vi "Elevator_Execute.vi"() -> ()   [LabVIEW 2019]
uses:
  Globals/Climb_Globals.vi
  <vilib>/Rock Robotics/WPI/ThirdParty/Phoenix-LabVIEW/Motor Controller/Controls/CTRE_Phoenix_MotorControl_ControlMode.ctl
  Globals/Sensor_Values.vi
  Globals/Solenoid Globals.vi
  <vilib>/Rock Robotics/WPI/Solenoid/WPI_SolenoidValue.ctl
  <vilib>/Rock Robotics/WPI/Solenoid/WPI_SolenoidSetEnum.vi
panel:
  in  "BrakeDelay(ms)":u32
  in  "acceptable_error":dbl
  out "Waveform Chart":dbl(graph)
  out "Left_Value_Added":dbl
  out "Right_Value_Added":dbl
  out "difference(left-right)":dbl
  out "Left_Side_Input":dbl
  out "Right_Side_Input":dbl
  in  "Left Down %V P-Gain":dbl=0.0003
  in  "Right Down %V P-Gain":dbl=0.0003
  in  "Left SpeedControl P-Gain":dbl
  in  "Right SpeedControl P-Gain":dbl
  in  "Max_Elevator_Speed":dbl
  in  "Left Up %V P-Gain":dbl=0.0003
  in  "Right Up %V P-Gain":dbl=0.0003
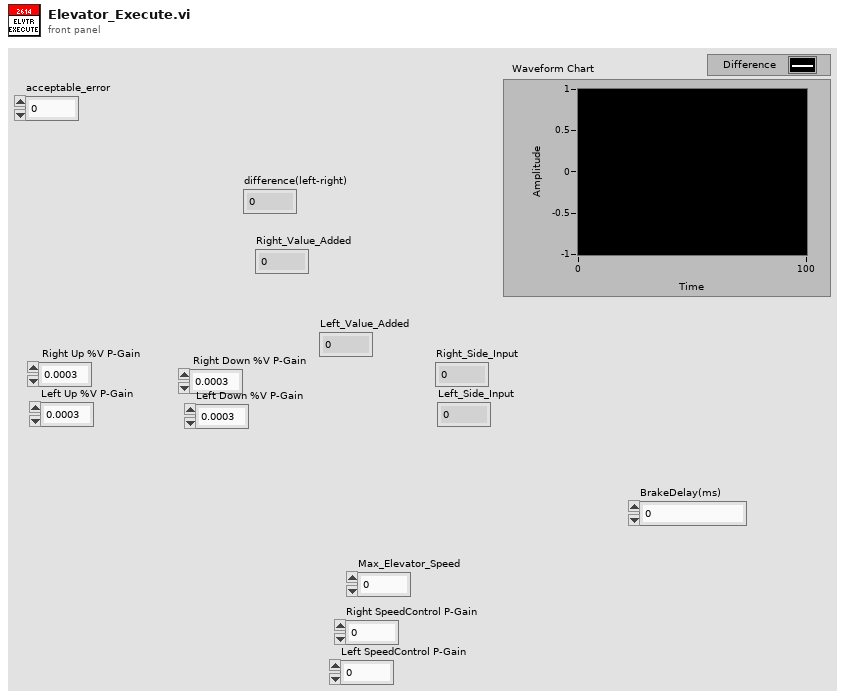
[diagram p1: front panel]
types:
  T1 = typedef "WPI_MotorControlDeviceRef.ctl" = cluster{"DeviceStatus":errorcluster, "Type":T2, "PWM":cluster{"PWM Channel":T3, "DeadBand":T4}, "CAN":cluster{"Device Number":u8, "SetOutput VI Ref":variant, "GetOutput VI Ref":variant, "Enable VI Ref":variant, "Disable VI Ref":variant, "Data":variant}, "Invert":bool, "DIO PWM":cluster{"PWM \"Enable\" Channel":T3, "DIOChannel":T5, "PWM Rate":dbl}}
  T2 = typedef "WPI_MotorControlType.ctl" = enum16{"PWM", "CAN", "DIO PWM"}
  T3 = typedef "FPGA_DIOPWMChannel.ctl" = enum8{"PWM 0", "PWM 1", "PWM 2", "PWM 3", "PWM 4", "PWM 5", "PWM 6", "PWM 7", "PWM 8", "PWM 9", "PWM MXP 0", "PWM MXP 1", "PWM MXP 2", "PWM MXP 3", "PWM MXP 4", "PWM MXP 5", "PWM MXP 6", "PWM MXP 7", "PWM MXP 8", "PWM MXP 9", "Invalid"}
  T4 = typedef "WPI_PWMDeadband.ctl" = cluster{"Name":string, "maxPositivePwm":i32, "minPositivePwm":i32, "centerPwm":i32, "maxNegativePwm":i32, "minNegativePwm":i32, "angularRange":u16}
  T5 = typedef "FPGA_DIOChannel.ctl" = enum8{"DIO 0", "DIO 1", "DIO 2", "DIO 3", "DIO 4", "DIO 5", "DIO 6", "DIO 7", "DIO 8", "DIO 9", "DIO MXP 0", "DIO MXP 1", "DIO MXP 2", "DIO MXP 3", "DIO MXP 4", "DIO MXP 5", "DIO MXP 6", "DIO MXP 7", "DIO MXP 8", "DIO MXP 9", "DIO MXP 10", "DIO MXP 11", "DIO MXP 12", "DIO MXP 13", "DIO MXP 14", "DIO MXP 15", "SPI Port CS1", "SPI Port CS2", "SPI Port CS3", "SPI Port MISO", "SPI Port MOSI", "Invalid"}
  T6 = typedef "WPI_SolenoidDevRef.ctl" = cluster{"DevStatus":errorcluster, "Pneumatics Control Module":u8, "Forward Solenoid Channel":T7, "Reverse Solenoid Channel":T7}
  T7 = typedef "WPI_SolenoidChannel.ctl" = enum8{"Solenoid 0", "Solenoid 1", "Solenoid 2", "Solenoid 3", "Solenoid 4", "Solenoid 5", "Solenoid 6", "Solenoid 7", "Invalid"}
  T8 = typedef "WPI_SolenoidValue.ctl" = enum16{"Off", "On", "Forward", "Reverse"}
  T9 = typedef "Climb_Elevator_Cluster.ctl" = cluster{"Extend?":bool, "Elevator_Throttle":dbl, "Control_States":T10}
  T10 = typedef "Climb_Elevator_Control_States.ctl" = enum16{"No-Op", "Brake", "Going_Up", "Going_Down", "Manual_PercentVoltage", "Manual_SpeedControl"}
  T11 = typedef "CTRE_Phoenix_MotorControl_ControlMode.ctl" = u16
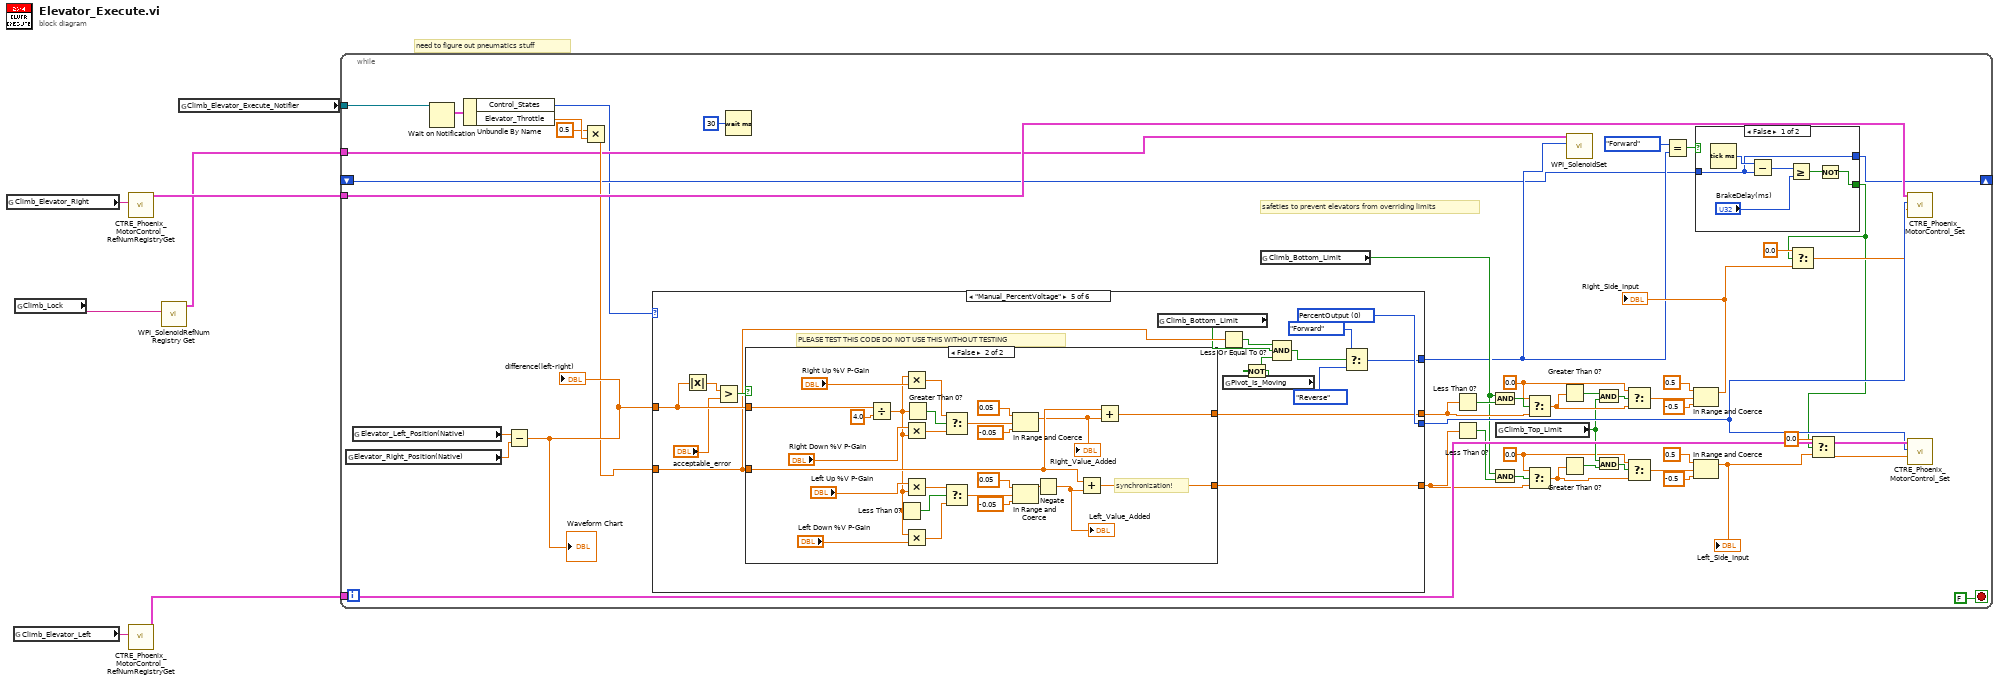
[diagram p0: block diagram]
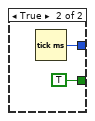
[diagram p2: hidden frame]
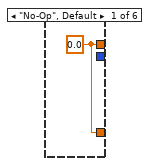
[diagram p3: hidden frame]
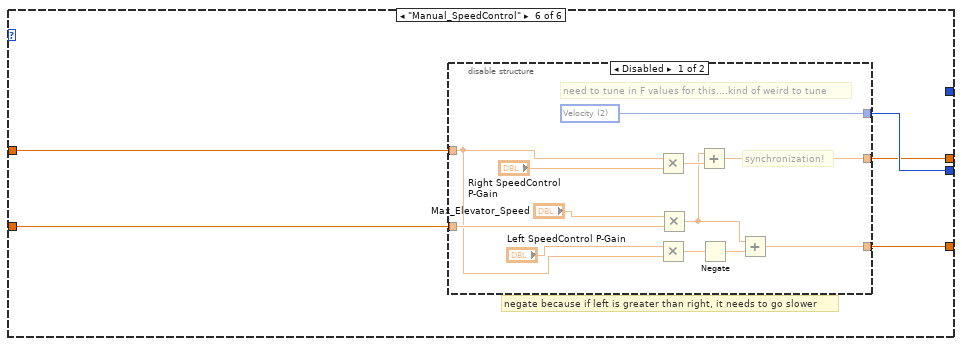
[diagram p8: hidden frame]
diagram:
  # "need to figure out pneumatics stuff"
  n1 = global read "Climb_Globals.vi" "Climb_Elevator_Right"() -> (w4:string)
  n2 = global read "Climb_Globals.vi" "Climb_Elevator_Left"() -> (w3:string)
  n3 = global read "Solenoid Globals.vi" "Climb_Lock"() -> (w2:string)
  n4 = call <vilib>:"CTRE_Phoenix_MotorControl_RefNumRegistryGet.vi"("refnum name"=w4) -> ("PhoenixMotorControlDevRef"=w6:T1)  [unwired: 9 in, 1 out]
  n5 = call <vilib>:"CTRE_Phoenix_MotorControl_RefNumRegistryGet.vi"("refnum name"=w3) -> ("PhoenixMotorControlDevRef"=w5:T1)  [unwired: 9 in, 1 out]
  n6 = call <vilib>:"WPI_SolenoidRefNum Registry Get.vi"("refnum name"=w2) -> ("SolenoidDevRef"=w1:T6)  [unwired: 9 in, 1 out]
  n7 = global read "Climb_Globals.vi" "Climb_Elevator_Execute_Notifier"() -> (w7:refnum<notifier>)
  n8 = while {
    tunnel: w7 -> [w55]
    tunnel: w6 -> [w53]
    tunnel: w5 -> [w54]
    tunnel: w1 -> [w21]
    shift-right: [w10] -> _
    shift-left: _ -> [w9]
    stop <- FALSE stop-if-true
    w37 = 0.0 ("t")
    w41 = 0.0 ("t")
    # "safeties to prevent elevators from overriding limits"
    n9 = global read "Sensor_Values.vi" "Elevator_Right_Position(Native)"() -> (w51:dbl)
    n10 = global read "Sensor_Values.vi" "Elevator_Left_Position(Native)"() -> (w50:dbl)
    n11 = Wait on Notification(notifier=w55) -> (notification=w25:T9)  [unwired: 3 in, 3 out]
    n12 = Unbundle By Name(w25) -> ("Control_States"=w8:T10, "Elevator_Throttle"=w24:dbl)
    n13 = Subtract(x=w50, y=w51) -> (x-y=w26:dbl)
    "difference(left-right)" <- w26
    "Waveform Chart" <- w26
    n14 = Multiply(x=0.5, y=w24) -> (x*y=w23:dbl)
    n15 = case shown="\"Manual_PercentVoltage\"" w8 {
      tunnel: w23 -> [_ _ _ _ w72 w111]
      tunnel: [_ _ _ _ w81 w112] -> w52
      tunnel: w26 -> [_ _ _ _ w78 w110]
      tunnel: [w65 _ _ _ w79 w108] -> w47
      tunnel: [w65 _ _ _ w80 w109] -> w29
      tunnel: [_ _ _ _ w74 _] -> w16
      frame "No-Op", Default {
        w65 = 0.0
      }
      frame "Brake" {
      }
      frame "Going_Up" {
      }
      frame "Going_Down" {
      }
      frame "Manual_PercentVoltage" {
        w81 = T11 0 items=["PercentOutput"=0, "Position"=1, "Velocity"=2, "Current"=3, "Follower"=5, "MotionProfile"=6, "MotionMagic"=7, "MotionProfileArc"=10, "Disabled"=15] ("Control Mode")
        # "PLEASE TEST THIS CODE DO NOT USE THIS WITHOUT TESTING"
        n16 = Absolute Value(x=w78) -> (abs(x)=w76:dbl)
        n17 = Greater?(x=w76, y="acceptable_error") -> (0:w77:bool)
        n18 = case shown="False" w77 {
          tunnel: w72 -> [w82 w106]
          tunnel: [w82 w104] -> w79
          tunnel: [w82 w103] -> w80
          tunnel: w78 -> [_ w96]
          frame True {
          }
          frame False {
            # "synchronization!"
            n19 = Divide(x=w96, y=4.0) -> (x/y=w83:dbl)
            n20 = Less Than 0?(x=w83) -> (x < 0?=w84:bool)
            n21 = Multiply(x=w83, y="Right Up %V P-Gain") -> (x*y=w91:dbl)
            n22 = Multiply(x="Right Down %V P-Gain", y=w83) -> (x*y=w90:dbl)
            n23 = Multiply(x="Left Up %V P-Gain", y=w83) -> (x*y=w87:dbl)
            n24 = Multiply(x=w83, y="Left Down %V P-Gain") -> (x*y=w86:dbl)
            n25 = Greater Than 0?(x=w83) -> (x > 0?=w92:bool)
            n26 = Select(t=w91, s=w92, f=w90) -> (s? t:f=w89:dbl)
            n27 = Select(t=w87, s=w84, f=w86) -> (s? t:f=w85:dbl)
            n28 = In Range and Coerce(upper limit=0.05, x=w89, lower limit=-0.05) -> (coerced(x)=w97:dbl)  [unwired: 1 out]
            "Right_Value_Added" <- w97
            n29 = In Range and Coerce(upper limit=0.05, x=w85, lower limit=-0.05) -> (coerced(x)=w99:dbl)  [unwired: 1 out]
            n30 = Negate(x=w99) -> (-x=w102:dbl)
            "Left_Value_Added" <- w102
            n31 = Add(x=w106, y=w102) -> (x+y=w103:dbl)
            n32 = Add(x=w106, y=w97) -> (x+y=w104:dbl)
          }
        }
        n33 = global read "Sensor_Values.vi" "Climb_Bottom_Limit"() -> (w70:bool)
        n34 = Less Or Equal To 0?(x=w72) -> (x <= 0?=w71:bool)
        n35 = global read "Climb_Globals.vi" "Pivot_Is_Moving"() -> (w67:bool)
        n36 = Not(x=w67) -> (.not. x?=w68:bool)
        n37 = Compound Arithmetic op=AND(w71, w70, w68) -> (w66:bool)
        n38 = Select(t=WPI_SolenoidValue."Forward" ("Value"), s=w66, f=WPI_SolenoidValue."Reverse" ("Value")) -> (s? t:f=w74:T8)
      }
      frame "Manual_SpeedControl" {
        # "negate because if left is greater than right, it needs to go slower"
        n39 = disable-structure shown="Disabled" {
          disable-tunnel: [w124 _] -> w112
          disable-tunnel: w111 -> [w123 _]
          disable-tunnel: w110 -> [w118 _]
          disable-tunnel: [w117 _] -> w109
          disable-tunnel: [w116 _] -> w108
          frame Disabled {
            w124 = T11 2 items=["PercentOutput"=0, "Position"=1, "Velocity"=2, "Current"=3, "Follower"=5, "MotionProfile"=6, "MotionMagic"=7, "MotionProfileArc"=10, "Disabled"=15] ("Control Mode")
            # "synchronization!"
            # "need to tune in F values for this....kind of weird to tune"
            n40 = Multiply(x=w118, y="Right SpeedControl P-Gain") -> (x*y=w121:dbl)
            n41 = Multiply(x="Left SpeedControl P-Gain", y=w118) -> (x*y=w120:dbl)
            n42 = Multiply(x="Max_Elevator_Speed", y=w123) -> (x*y=w115:dbl)
            n43 = Add(x=w115, y=w121) -> (x+y=w116:dbl)
            n44 = Negate(x=w120) -> (-x=w119:dbl)
            n45 = Add(x=w115, y=w119) -> (x+y=w117:dbl)
          }
          frame Enabled {
          }
        }
      }
    }
    n46 = Wait (ms)(milliseconds to wait=u32 30) -> ()  [unwired: 1 out]
    n47 = global read "Sensor_Values.vi" "Climb_Bottom_Limit"() -> (w45:bool)
    n48 = Less Than 0?(x=w47) -> (x < 0?=w49:bool)
    n49 = Less Than 0?(x=w29) -> (x < 0?=w28:bool)
    n50 = And(x=w45, y=w49) -> (x .and. y?=w48:bool)
    n51 = And(x=w45, y=w28) -> (x .and. y?=w46:bool)
    n52 = global read "Sensor_Values.vi" "Climb_Top_Limit"() -> (w39:bool)
    n53 = Select(t=w41, s=w48, f=w47) -> (s? t:f=w42:dbl)
    n54 = Select(t=w37, s=w46, f=w29) -> (s? t:f=w36:dbl)
    n55 = Greater Than 0?(x=w42) -> (x > 0?=w43:bool)
    n56 = Greater Than 0?(x=w36) -> (x > 0?=w38:bool)
    n57 = call-poly <vilib>:"WPI_SolenoidSet.vi"("Value"=w16, "SolenoidDevRef"=w21) -> ()  [unwired: 8 in, 2 out]
    n58 = And(x=w43, y=w39) -> (x .and. y?=w44:bool)
    n59 = And(x=w39, y=w38) -> (x .and. y?=w40:bool)
    n60 = Select(t=w41, s=w44, f=w42) -> (s? t:f=w30:dbl)
    n61 = Select(t=w37, s=w40, f=w36) -> (s? t:f=w35:dbl)
    n62 = Equal?(x=WPI_SolenoidValue."Forward", y=w16) -> (x = y?=w12:bool)
    n63 = In Range and Coerce(upper limit=0.5, x=w30, lower limit=-0.5) -> (coerced(x)=w20:dbl)  [unwired: 1 out]
    "Right_Side_Input" <- w20
    n64 = In Range and Coerce(upper limit=0.5, x=w35, lower limit=-0.5) -> (coerced(x)=w18:dbl)  [unwired: 1 out]
    "Left_Side_Input" <- w18
    n65 = case shown="False" w12 {
      tunnel: [w57 TRUE] -> w11
      tunnel: [w61 w63] -> w10
      tunnel: w9 -> [w61 _]
      frame False {
        n66 = Tick Count (ms)() -> (millisecond timer value=w62:u32)
        n67 = Subtract(x=w62, y=w61) -> (x-y=w60:u32)
        n68 = Greater Or Equal?(x=w60, y="BrakeDelay(ms)") -> (x >= y?=w58:bool)
        n69 = Not(x=w58) -> (.not. x?=w57:bool)
      }
      frame True {
        n70 = Tick Count (ms)() -> (millisecond timer value=w63:u32)
      }
    }
    n71 = Select(t=0.0, s=w11, f=w20) -> (s? t:f=w19:dbl)
    n72 = Select(t=0.0, s=w11, f=w18) -> (s? t:f=w17:dbl)
    n73 = call <vilib>:"CTRE_Phoenix_MotorControl_Set.vi"("Output"=w19, "Control Mode"=w52, "PhoenixMotorControlDevRef"=w53) -> ()  [unwired: 7 in, 2 out]
    n74 = call <vilib>:"CTRE_Phoenix_MotorControl_Set.vi"("Output"=w17, "Control Mode"=w52, "PhoenixMotorControlDevRef"=w54) -> ()  [unwired: 7 in, 2 out]
  }
